vi "newCameraPrompt.vi"(11 "DeviceList":string[](array[string])) -> (1 "valid":bool, 2 "ontrakOut":i32, 3 "DeviceOut":string)   [LabVIEW 2013]
panel:
  in  "Ontrak":bool
  in  "Ontrak Channel":i32
  in  "cancelButton":bool
  in  "okButton":bool
  in  "Device":string(combo)
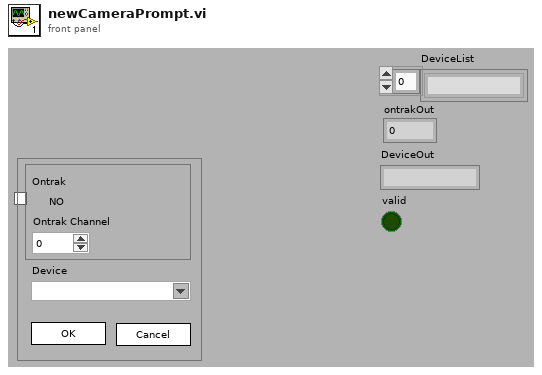
[diagram p1: front panel]
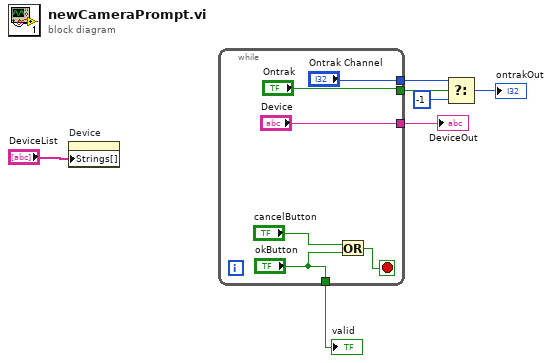
[diagram p0: block diagram]
diagram:
  n1 = property on="Device" class="CmbBox"("Strings[]"="DeviceList") -> ()  [unwired: 2 in, 2 out]
  n2 = while {
    tunnel: ["okButton"] -> w6
    tunnel: ["Ontrak"] -> w4
    tunnel: ["Ontrak Channel"] -> w3
    tunnel: ["Device"] -> w1
    stop <- w12 stop-if-true
    n3 = Or(x="cancelButton", y="okButton") -> (x .or. y?=w12:bool)
  }
  "DeviceOut" <- w1
  "valid" <- w6
  n4 = Select(t=w3, s=w4, f=-1) -> (s? t:f=→"ontrakOut":i32)
